vi "Highlight Selected Color.vi"(8 "error in (no error)":errorcluster, 10 "Selected Color":u32(colorbox), 11 "ColorSelector in":refnum<class "ColorSelector.lvclass">) -> (0 "error out":errorcluster, 3 "ColorSelector (dup)":refnum<class "ColorSelector.lvclass">)   [LabVIEW 2015, in "ColorSelector.lvclass"]
doc: "This VI draws the crosshairs on the correct coordinate in the Color Selector.\n<b> </b> <b> </b>\n©2017 Q Software Innovations, LLC (QSI)\nwritten by Quentin Alldredge\nproduced in LabVIEW 2015\n\nsupport@qsoftwareinnovations.com\nwww.qsoftwareinnovations.com\n\nAll rights reserved.\n\nRedistribution and use in source and binary forms, with or without modification, are permitted provided that the following conditions are met:\n\n * Redistributions of source code must retain the above copyright notice, this list of conditions and the following disclaimer.\n * Redistributions in binary form must reproduce the above copyright notice, this list of conditions and the following disclaimer in the documentation and/or other materials provided with the distribution.\n * Neither the name of Q Software Innovations, LLC. nor the names of its contributors may be used to endorse or promote products derived from this software without specific prior written permission.\n\nTHIS SOFTWARE IS PROVIDED BY THE COPYRIGHT HOLDERS AND CONTRIBUTORS \"AS IS\" AND ANY EXPRESS OR IMPLIED WARRANTIES, INCLUDING, BUT NOT LIMITED TO, THE IMPLIED WARRANTIES OF MERCHANTABILITY AND FITNESS FOR A PARTICULAR PURPOSE ARE DISCLAIMED. IN NO EVENT SHALL THE COPYRIGHT OWNER OR CONTRIBUTORS BE LIABLE FOR ANY DIRECT, INDIRECT, INCIDENTAL, SPECIAL, EXEMPLARY, OR CONSEQUENTIAL DAMAGES (INCLUDING, BUT NOT LIMITED TO, PROCUREMENT OF SUBSTITUTE GOODS OR SERVICES; LOSS OF USE, DATA, OR PROFITS; OR BUSINESS INTERRUPTION) HOWEVER CAUSED AND ON ANY THEORY OF LIABILITY, WHETHER IN CONTRACT, STRICT LIABILITY, OR TORT (INCLUDING NEGLIGENCE OR OTHERWISE) ARISING IN ANY WAY OUT OF THE USE OF THIS SOFTWARE, EVEN IF ADVISED OF THE POSSIBILITY OF SUCH DAMAGE."
uses:
  ColorSelector.lvclass
  ColorSelector.lvclass/ColorSelector.ctl
  Read ColorSelectPic.vi
  Read ColorGridCoords.vi
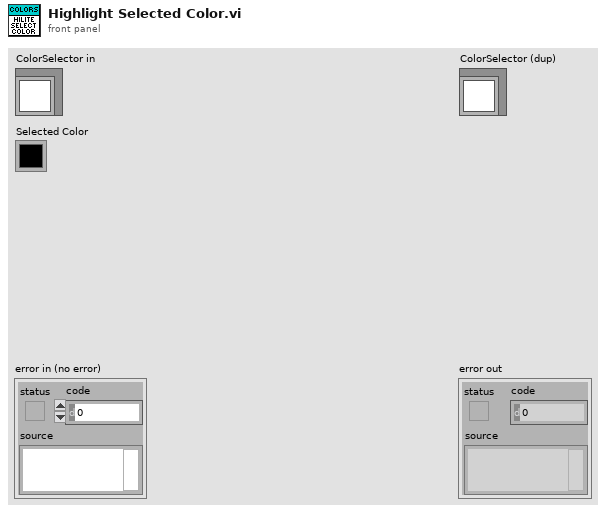
[diagram p1: front panel]
types:
  T1 = cluster{"Width":i16, "Style":enum32{"Solid", "Dash", "Dot", "DashDot", "DashDotDot"}}
  T2 = cluster{"left":i16, "top":i16, "right":i16, "bottom":i16}
  T3 = typedef "LVPoint32TypeDef.ctl" = cluster{"Horizontal":i32, "Vertical":i32}
  T4 = typedef "imagedata.ctl" = cluster{"image type":i32, "image depth":i32, "image":u8[], "mask":u8[], "colors":u32[], "Rectangle":cluster{"left":i16, "top":i16, "right":i16, "bottom":i16}}
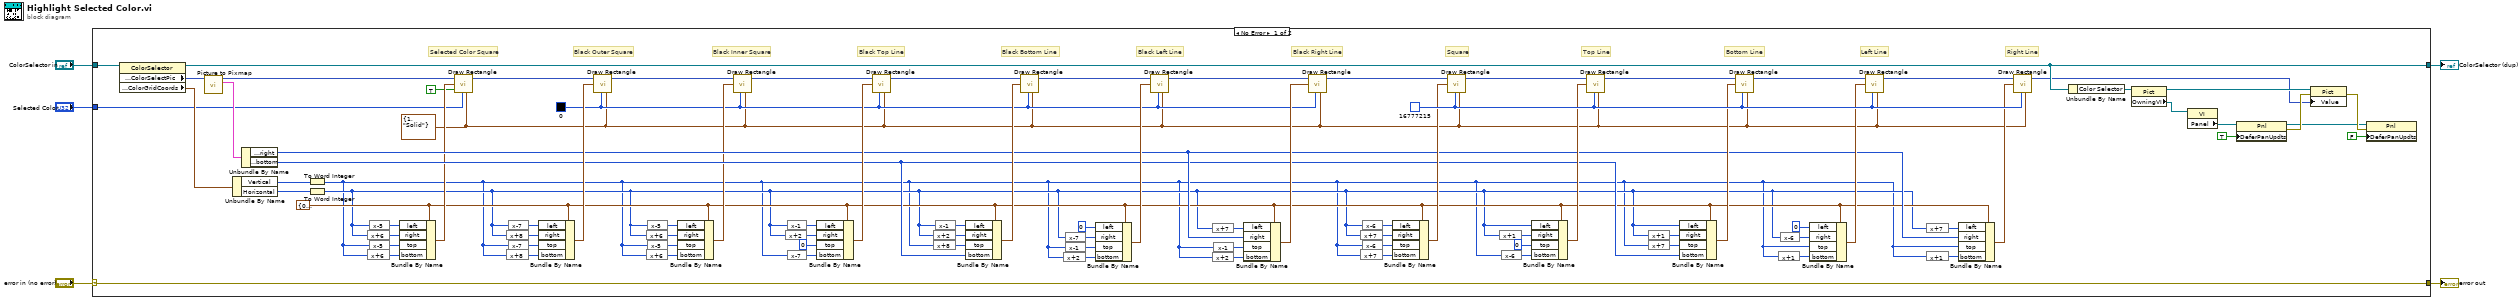
[diagram p0: block diagram]
diagram:
  n1 = case shown="No Error" "error in (no error)" {
    selector: "error in (no error)" -> [w97 w99]
    tunnel: [w97 w99] -> w4
    tunnel: [w76 w98] -> w2
    tunnel: "ColorSelector in" -> [w78 w98]
    tunnel: "Selected Color" -> [w7 _]
    frame No Error {
      w46 = u32 16777215 ("color(black)")
      w23 = u32 0 ("color(black)")
      w8 = T1 {"Width"=1, "Style"=enum."Solid"} ("pen")
      w11 = T2 {"left"=0, "top"=0, "right"=0, "bottom"=0} ("rect")
      # "Selected Color Square"
      # "Black Inner Square"
      # "Right Line"
      # "Left Line"
      # "Bottom Line"
      # "Top Line"
      # "Square"
      # "Black Right Line"
      # "Black Left Line"
      # "Black Bottom Line"
      # "Black Top Line"
      # "Black Outer Square"
      n2 = property class="ColorSelector"(reference=w78) -> (reference out=w76:refnum<class "ColorSelector.lvclass">, "State Data:Accessors:ColorSelectPic"=w96:picture, "State Data:Accessors:ColorGridCoords"=w75:T3)  [unwired: 1 in, 1 out]
      n3 = call <vilib>:"Picture to Pixmap.vi"("picture"=w96) -> ("image data"=w92:T4, "new picture"=w13:picture)  [unwired: 9 in]
      n4 = Unbundle By Name(w75) -> ("Vertical"=w73:i32, "Horizontal"=w71:i32)
      n5 = Unbundle By Name(w92) -> ("Rectangle.right"=w32:i16, "Rectangle.bottom"=w31:i16)
      n6 = To Word Integer(number=w73) -> (16bit integer=w9:i16)
      n7 = To Word Integer(number=w71) -> (16bit integer=w10:i16)
      n8 = expression code="x+6"(w10) -> (w14:i16)
      n9 = expression code="x+6"(w9) -> (w16:i16)
      n10 = expression code="x-5"(w10) -> (w15:i16)
      n11 = expression code="x-5"(w9) -> (w17:i16)
      n12 = Bundle By Name(cluster=w11, "left"=w15, "right"=w14, "top"=w17, "bottom"=w16) -> (w18:T2)
      n13 = call <vilib>:"Draw Rectangle.vi"("picture"=w13, "rect"=w18, "fill?(F)"=TRUE, "color(black)"=w7, "pen"=w8) -> ("new picture"=w12:picture)  [unwired: 4 in]
      n14 = expression code="x+8"(w10) -> (w69:i16)
      n15 = expression code="x+8"(w9) -> (w72:i16)
      n16 = expression code="x-7"(w10) -> (w70:i16)
      n17 = expression code="x-7"(w9) -> (w74:i16)
      n18 = Bundle By Name(cluster=w11, "left"=w70, "right"=w69, "top"=w74, "bottom"=w72) -> (w95:T2)
      n19 = call <vilib>:"Draw Rectangle.vi"("picture"=w12, "rect"=w95, "color(black)"=w23, "pen"=w8) -> ("new picture"=w25:picture)  [unwired: 5 in]
      n20 = expression code="x+6"(w10) -> (w30:i16)
      n21 = expression code="x+6"(w9) -> (w28:i16)
      n22 = expression code="x-5"(w10) -> (w29:i16)
      n23 = expression code="x-5"(w9) -> (w27:i16)
      n24 = Bundle By Name(cluster=w11, "left"=w29, "right"=w30, "top"=w27, "bottom"=w28) -> (w26:T2)
      n25 = call <vilib>:"Draw Rectangle.vi"("picture"=w25, "rect"=w26, "color(black)"=w23, "pen"=w8) -> ("new picture"=w24:picture)  [unwired: 5 in]
      n26 = expression code="x+2"(w10) -> (w68:i16)
      n27 = expression code="x-1"(w10) -> (w22:i16)
      n28 = expression code="x-7"(w9) -> (w66:i16)
      n29 = Bundle By Name(cluster=w11, "left"=w22, "right"=w68, "top"=i16 0, "bottom"=w66) -> (w94:T2)
      n30 = call <vilib>:"Draw Rectangle.vi"("picture"=w24, "rect"=w94, "color(black)"=w23, "pen"=w8) -> ("new picture"=w93:picture)  [unwired: 5 in]
      n31 = expression code="x+2"(w10) -> (w65:i16)
      n32 = expression code="x+8"(w9) -> (w64:i16)
      n33 = expression code="x-1"(w10) -> (w21:i16)
      n34 = Bundle By Name(cluster=w11, "left"=w21, "right"=w65, "top"=w64, "bottom"=w31) -> (w91:T2)
      n35 = call <vilib>:"Draw Rectangle.vi"("picture"=w93, "rect"=w91, "color(black)"=w23, "pen"=w8) -> ("new picture"=w90:picture)  [unwired: 5 in]
      n36 = expression code="x+2"(w9) -> (w61:i16)
      n37 = expression code="x-7"(w10) -> (w62:i16)
      n38 = expression code="x-1"(w9) -> (w20:i16)
      n39 = Bundle By Name(cluster=w11, "left"=i16 0, "right"=w62, "top"=w20, "bottom"=w61) -> (w89:T2)
      n40 = call <vilib>:"Draw Rectangle.vi"("picture"=w90, "rect"=w89, "color(black)"=w23, "pen"=w8) -> ("new picture"=w88:picture)  [unwired: 5 in]
      n41 = expression code="x+7"(w10) -> (w60:i16)
      n42 = expression code="x+2"(w9) -> (w59:i16)
      n43 = expression code="x-1"(w9) -> (w19:i16)
      n44 = Bundle By Name(cluster=w11, "left"=w60, "right"=w32, "top"=w19, "bottom"=w59) -> (w87:T2)
      n45 = call <vilib>:"Draw Rectangle.vi"("picture"=w88, "rect"=w87, "color(black)"=w23, "pen"=w8) -> ("new picture"=w34:picture)  [unwired: 5 in]
      n46 = expression code="x+7"(w10) -> (w48:i16)
      n47 = expression code="x+7"(w9) -> (w45:i16)
      n48 = expression code="x-6"(w10) -> (w47:i16)
      n49 = expression code="x-6"(w9) -> (w44:i16)
      n50 = Bundle By Name(cluster=w11, "left"=w47, "right"=w48, "top"=w44, "bottom"=w45) -> (w35:T2)
      n51 = call <vilib>:"Draw Rectangle.vi"("picture"=w34, "rect"=w35, "color(black)"=w46, "pen"=w8) -> ("new picture"=w36:picture)  [unwired: 5 in]
      n52 = expression code="x+1"(w10) -> (w49:i16)
      n53 = expression code="x-6"(w9) -> (w51:i16)
      n54 = Bundle By Name(cluster=w11, "left"=w10, "right"=w49, "top"=i16 0, "bottom"=w51) -> (w37:T2)
      n55 = call <vilib>:"Draw Rectangle.vi"("picture"=w36, "rect"=w37, "color(black)"=w46, "pen"=w8) -> ("new picture"=w38:picture)  [unwired: 5 in]
      n56 = expression code="x+1"(w10) -> (w52:i16)
      n57 = expression code="x+7"(w9) -> (w53:i16)
      n58 = Bundle By Name(cluster=w11, "left"=w10, "right"=w52, "top"=w53, "bottom"=w31) -> (w39:T2)
      n59 = call <vilib>:"Draw Rectangle.vi"("picture"=w38, "rect"=w39, "color(black)"=w46, "pen"=w8) -> ("new picture"=w40:picture)  [unwired: 5 in]
      n60 = expression code="x+1"(w9) -> (w56:i16)
      n61 = expression code="x-6"(w10) -> (w55:i16)
      n62 = Bundle By Name(cluster=w11, "left"=i16 0, "right"=w55, "top"=w9, "bottom"=w56) -> (w41:T2)
      n63 = call <vilib>:"Draw Rectangle.vi"("picture"=w40, "rect"=w41, "color(black)"=w46, "pen"=w8) -> ("new picture"=w42:picture)  [unwired: 5 in]
      n64 = expression code="x+7"(w10) -> (w57:i16)
      n65 = expression code="x+1"(w9) -> (w58:i16)
      n66 = Bundle By Name(cluster=w11, "left"=w57, "right"=w32, "top"=w9, "bottom"=w58) -> (w43:T2)
      n67 = call <vilib>:"Draw Rectangle.vi"("picture"=w42, "rect"=w43, "color(black)"=w46, "pen"=w8) -> ("new picture"=w33:picture)  [unwired: 5 in]
      n68 = Unbundle By Name(w76) -> ("Color Selector"=w77:refnum<vi>)
      n69 = property class="Pict"(reference=w77) -> (reference out=w86:refnum<vi>, "OwningVI"=w85:refnum<vi>)  [unwired: 1 in, 1 out]
      n70 = property class="VI"(reference=w85) -> ("Panel"=w84:refnum<vi>)  [unwired: 1 in, 2 out]
      n71 = property class="Pnl"(reference=w84, "DeferPanUpdts"=TRUE ("Defer Panel Updates")) -> (reference out=w80:refnum<vi>, error out=w82:errorcluster)  [unwired: 1 in]
      n72 = property on="Property Node" class="Pict"(reference=w86, error in=w82, "Value"=w33) -> (error out=w81:errorcluster)  [unwired: 1 out]
      n73 = property class="Pnl"(reference=w80, error in=w81, "DeferPanUpdts"=FALSE ("Defer Panel Updates")) -> ()  [unwired: 2 out]
    }
    frame Error {
    }
  }
  "error out" <- w4
  "ColorSelector (dup)" <- w2
